vi "Example 01 - Basic Stack Manipulation.vi"() -> ()   [LabVIEW 2020]
uses:
  Lua for LabVIEW/Lua/Lua.lvclass
panel:
  out "Stack F (empty)":string[](array[string])
  out "Stack E":string[](array[string])
  out "Stack D":string[](array[string])
  out "Stack C":string[](array[string])
  out "Stack B":string[](array[string])
  out "Stack A":string[](array[string])
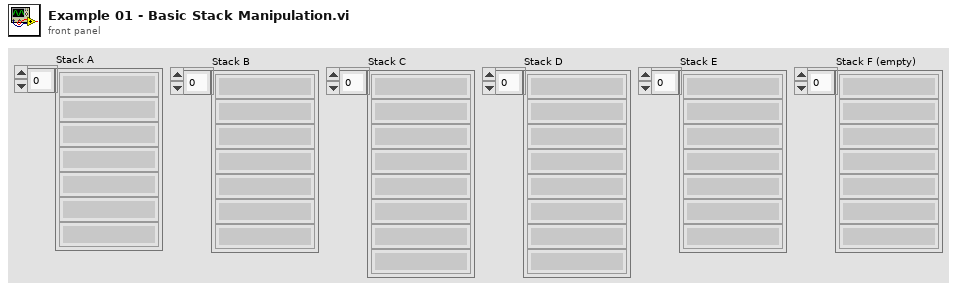
[diagram p1: front panel]
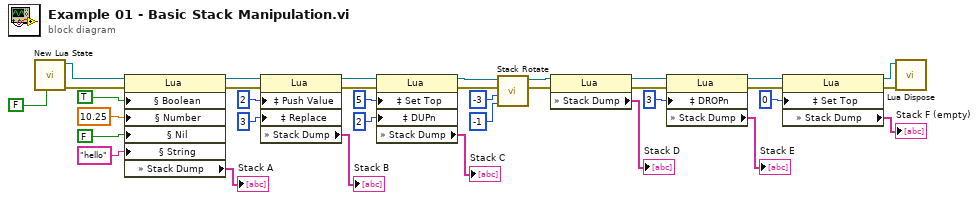
[diagram p0: block diagram]
diagram:
  n1 = call "New Lua State.vi"("open libs? (T)"=FALSE) -> ("error out"=w33:errorcluster, "Lua out"=w35:refnum<class "Lua.lvclass">)  [unwired: 9 in]
  n2 = property class="Lua"(reference=w35, error in=w33, "§ Boolean"=TRUE ("Push Boolean"), "§ Number"=10.25 ("Push Number"), "§ Nil"=FALSE ("Push Nil"), "§ String"="hello" ("Push String")) -> (reference out=w34:refnum<class "Lua.lvclass">, error out=w27:errorcluster, "» Stack Dump"=→"Stack A":string[])
  n3 = property class="Lua"(reference=w34, error in=w27, "‡ Push Value"=2 ("(Stack) Replace"), "‡ Replace"=3 ("(Stack) Replace")) -> (reference out=w23:refnum<class "Lua.lvclass">, error out=w22:errorcluster, "» Stack Dump"=→"Stack B":string[])
  n4 = property class="Lua"(reference=w23, error in=w22, "‡ Set Top"=5 ("(Stack) Set Top"), "‡ DUPn"=2) -> (reference out=w3:refnum<class "Lua.lvclass">, error out=w4:errorcluster, "» Stack Dump"=→"Stack C":string[])
  n5 = call-dynamic "Stack Rotate.vi"("n"=-1, "index"=-3, "error in (no error)"=w4, "Lua in"=w3) -> ("error out"=w5:errorcluster, "Lua out"=w6:refnum<class "Lua.lvclass">)  [unwired: 6 in]
  n6 = property class="Lua"(reference=w6, error in=w5) -> (reference out=w18:refnum<class "Lua.lvclass">, error out=w9:errorcluster, "» Stack Dump"=→"Stack D":string[])
  n7 = property class="Lua"(reference=w18, error in=w9, "‡ DROPn"=3 ("(Stack) Remove")) -> (reference out=w15:refnum<class "Lua.lvclass">, error out=w10:errorcluster, "» Stack Dump"=→"Stack E":string[])
  n8 = property class="Lua"(reference=w15, error in=w10, "‡ Set Top"=0 ("(Stack) Set Top")) -> (reference out=w11:refnum<class "Lua.lvclass">, error out=w12:errorcluster, "» Stack Dump"=→"Stack F (empty)":string[])
  n9 = call-dynamic "Lua Dispose.vi"("error in (no error)"=w12, "Lua in"=w11) -> ()  [unwired: 9 in, 1 out]
